vi "EEPROM Read.vi"   [LabVIEW 2014]
uses:
  QwaveSys_ESP8266/QwaveSys_ESP8266.lvlib
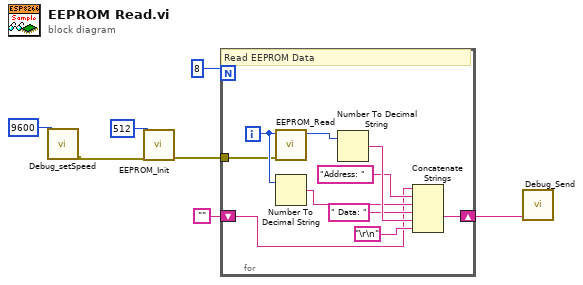
[diagram p0: block diagram]
diagram:
  n1 = call "Debug_setSpeed.vi"("Speed"=u32 9600) -> ("error out"=w3:errorcluster)  [unwired: 10 in]
  n2 = call "EEPROM_Init.vi"("error in (no error)"=w3, "size (4-4096 bytes)"=u16 512) -> ("error out"=w4:errorcluster)  [unwired: 9 in]
  n3 = for {
    N: 8 -> [_]
    tunnel: w4 -> [w8]
    shift-right: [w15] -> w1
    shift-left: "" -> [w9]
    i -> [w13]
    # "Read EEPROM Data"
    n4 = call "EEPROM_Read.vi"("error in (no error)"=w8, "Address"=w13) -> ("Data"=w17:u8)  [unwired: 8 in, 1 out]
    n5 = Number To Decimal String(number=w13) -> (decimal integer string=w12:string)  [unwired: 1 in]
    n6 = Number To Decimal String(number=w17) -> (decimal integer string=w16:string)  [unwired: 1 in]
    n7 = Concatenate Strings(w9, "Address: " ("string"), w12, " Data: " ("string"), w16, "\r\n") -> (w15:string)
  }
  n8 = call "Debug_Send.vi"("DATA"=w1) -> ()  [unwired: 11 in]
